vi "WristEncoderToAngle.vi"(9 "ElbowAngle":dbl, 10 "ShoulderAngle":dbl, 11 "encoderPulses":i32) -> (2 "Theta4":dbl, 3 "wrist angle(deg)":dbl)   [LabVIEW 2018]
uses:
  Arm Constants.vi
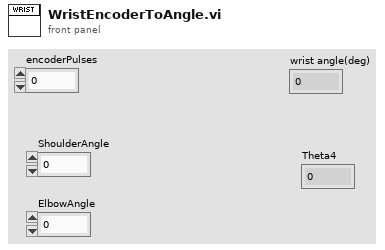
[diagram p1: front panel]
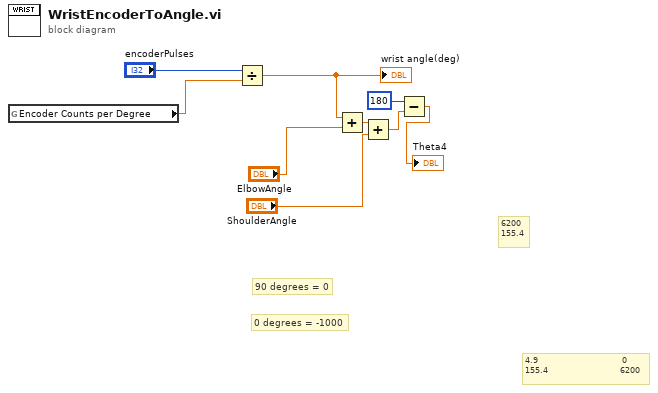
[diagram p0: block diagram]
diagram:
  # "4.9                            0\n155.4                        6200"
  # "6200\n155.4"
  # "0 degrees = -1000"
  # "90 degrees = 0"
  n1 = global read "Arm Constants.vi" "Encoder Counts per Degree"() -> (w4:dbl)
  n2 = Divide(x="encoderPulses", y=w4) -> (x/y=w8:dbl)
  "wrist angle(deg)" <- w8
  n3 = Add(x=w8, y="ElbowAngle") -> (x+y=w6:dbl)
  n4 = Add(x=w6, y="ShoulderAngle") -> (x+y=w2:dbl)
  n5 = Subtract(x=180, y=w2) -> (x-y=→"Theta4":dbl)
